vi "GetType.vi"(8 "error in (no error)":errorcluster, 11 "Polling Interval Msg":refnum<class "Polling Interval Msg.lvclass">) -> (0 "error out":errorcluster, 2 "Data Sample":variant, 3 "Polling Interval Msg":refnum<class "Polling Interval Msg.lvclass">)   [LabVIEW 2015, in "CS++BaseActor.lvlib" / "Polling Interval Msg.lvclass"]
uses:
  Polling Interval Msg.lvclass
  Polling Interval Msg.lvclass/Polling Interval Msg.ctl
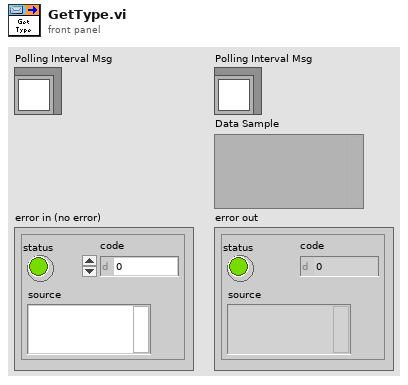
[diagram p1: front panel]
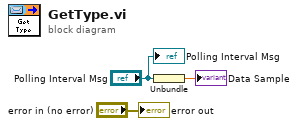
[diagram p0: block diagram]
diagram:
  n1 = Unbundle("Polling Interval Msg") -> (→"Data Sample":dbl[unit])
  "error out" <- "error in (no error)"
  "Polling Interval Msg" <- "Polling Interval Msg"
